vi "WriteHeaders.vi"(8 "error in":errorcluster, 9 "Date and Time":string, 10 "Match Number":dbl, 11 "refnum in":refnum<file>) -> (0 "error out":errorcluster, 3 "refnum out":refnum<file>)   [LabVIEW 2016]
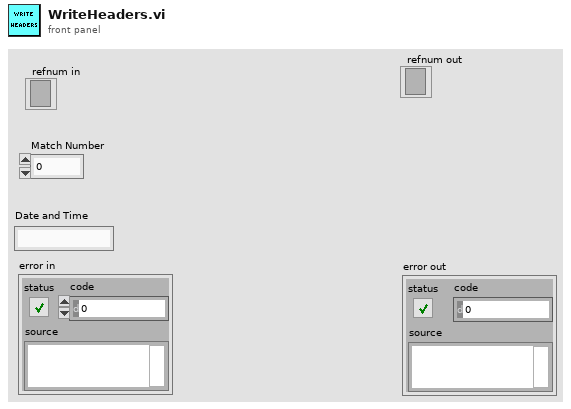
[diagram p1: front panel]
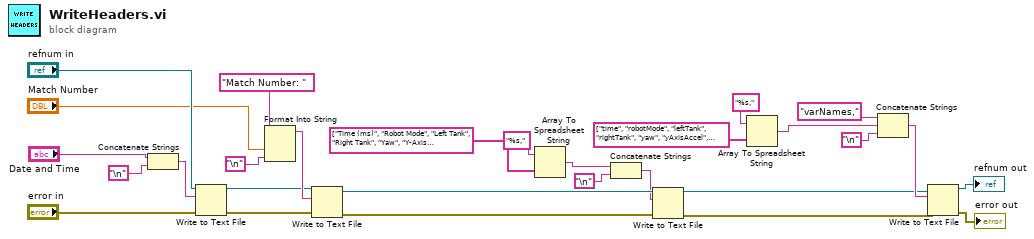
[diagram p0: block diagram]
diagram:
  n1 = Concatenate Strings("Date and Time", "\n") -> (w26:string)
  n2 = Write to Text File(file (use dialog)="refnum in", text=w26, error in="error in") -> (refnum out=w19:refnum<file>, error out=w18:errorcluster)  [unwired: 1 in, 1 out]
  n3 = Format Into String(initial string="Match Number: ", "Match Number", "\n") -> (resulting string=w20:string)  [unwired: 2 in, 1 out]
  n4 = Write to Text File(file (use dialog)=w19, text=w20, error in=w18) -> (refnum out=w17:refnum<file>, error out=w14:errorcluster)  [unwired: 1 in, 1 out]
  n5 = Array To Spreadsheet String(array=string[] ["Time (ms)", "Robot Mode", "Left Tank", "Right Tank", "Yaw", "Y-Axis Acceleration", "Moving?", "Left Distance", "Right Distance", "Left Velocity", "Right Velocity", "PWM 0 PDP 2 (L Drive)", "PWM 1 PDP 4", "PWM 2 PDP 1", "PWM 3 PDP 0 (L Drive)", "PWM 4 PDP 15 (L Drive)", "PWM 5 PDP 12 (R Drive)", "PWM 6 PDP 13 (R Drive)", "PWM 7 PDP 14 (R Drive)", "Voltage"], 3:"%s," ("format string")) -> (spreadsheet string=w11:string)  [unwired: 1 in]
  n6 = Concatenate Strings(w11, "\n") -> (w1:string)
  n7 = Write to Text File(file (use dialog)=w17, text=w1, error in=w14) -> (refnum out=w5:refnum<file>, error out=w4:errorcluster)  [unwired: 1 in, 1 out]
  n8 = Array To Spreadsheet String(array=string[] ["time", "robotMode", "leftTank", "rightTank", "yaw", "yAxisAccel", "isMoving", "leftDistance", "rightDistance", "leftVelocity", "rightVelocity", "PDP2", "PDP4", "PDP1", "PDP0", "PDP15", "PDP12", "PDP13", "PDP14", "voltage"], 3:"%s," ("format string")) -> (spreadsheet string=w7:string)  [unwired: 1 in]
  n9 = Concatenate Strings("varNames," ("string"), w7, "\n") -> (w6:string)
  n10 = Write to Text File(file (use dialog)=w5, text=w6, error in=w4) -> (refnum out=→"refnum out":refnum<file>, error out=→"error out":errorcluster)  [unwired: 1 in, 1 out]
